vi "N6700_Clear_OVP_and_OCP.vi"(6 "Delay (ms)":u32=100, 7 "Channels (1:4)":i32[](array[numeric])=[1, 2, 3, 4], 8 "error in (no error)":errorcluster {"code" format="%.0x"}, 11 "VISA resource name":refnum<visa-resource-name>) -> (0 "error out":errorcluster {"code" format="%.0x"}, 3 "VISA resource name out":refnum<visa-resource-name>)   [LabVIEW 2015]
doc: "This VI takes a measurement on the output signal and returns the measured value."
uses:
  <instrlib>/Agilent N6700 Series/Agilent N6700 Series.lvlib
panel:
  # "Note: Delete array element for empty channels"
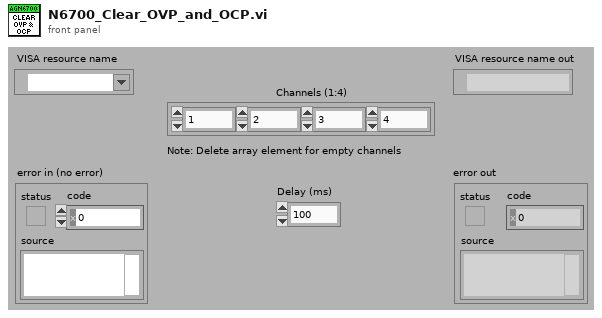
[diagram p1: front panel]
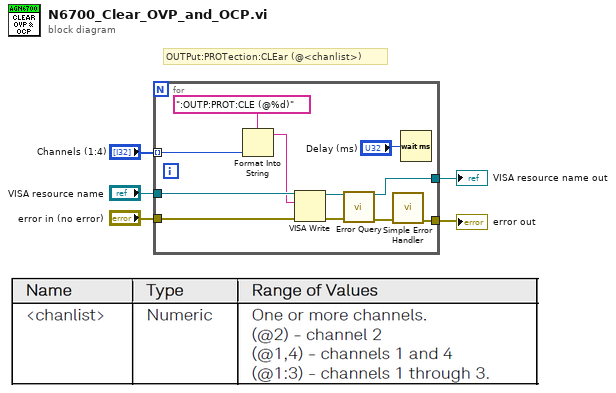
[diagram p0: block diagram]
diagram:
  # "OUTPut:PROTection:CLEar (@<chanlist>)"
  n1 = for {
    tunnel: "Channels (1:4)" -> [w15] mode=indexing
    tunnel: [w12] -> w4
    tunnel: "VISA resource name" -> [w11]
    tunnel: "error in (no error)" -> [w10]
    tunnel: [w6] -> w1
    n2 = Format Into String(format string=":OUTP:PROT:CLE (@%d)", w15) -> (resulting string=w9:string)  [unwired: 2 in, 1 out]
    n3 = VISA Write(VISA resource name=w11, write buffer=w9, error in (no error)=w10) -> (VISA resource name out=w14:refnum<visa-resource-name>, error out=w13:errorcluster)  [unwired: 1 out]
    n4 = call <instrlib>:"Error Query.vi"("VISA resource name"=w14, "error in (no error)"=w13) -> ("VISA resource name out"=w12:refnum<visa-resource-name>, "error out"=w7:errorcluster)  [unwired: 10 in, 2 out]
    n5 = call <vilib>:"Simple Error Handler.vi"("error in (no error)"=w7) -> ("error out"=w6:errorcluster)  [unwired: 4 in, 4 out]
    n6 = Wait (ms)(milliseconds to wait="Delay (ms)") -> ()  [unwired: 1 out]
  }
  "error out" <- w1
  "VISA resource name out" <- w4
